vi "Send command.vi"(3 "Value":u16, 4 "Command":T1=17 items=["Measured main TEC temperature"=0, "Measured SHG heater temperature"=1, "Measured BRF heater temperature"=2, "Main TEC temperature command"=3, "SHG heater temperature command"=4, "BRF heater temperature command"=5, "Main TEC drive"=6, "SHG heater drive"=7, "BRF heater drive"=8, "Output power from photodiode"=9, "Output power setpoint (Get)"=10, "Output power setpoint (Set)"=11, "Start-up power setting (Get)"=12, "Start-up power setting (Set)"=13, "Measured LDD current"=14, "Maximum LDD current limit"=15, "16-bit fault code"=16, "Head serial number"=17, "Head board rev"=18, "Head type"=19, "LDD enable state"=20, "Key switch command (Get)"=24, "Key switch command (Set)"=25, "Key switch actual"=26, "Interlock status"=27, "Head hours"=28, "Photo or current mode command (Get)"=29, "Photo or current mode command (Set)"=30, "Photo or current mode actual"=31, "Analog input enable command (Get)"=32, "Analog input enable command (Set)"=33, "Analog input actual"=34, "Power supply glue input"=36, "Power supply glue output"=37], 5 "Device handle":u32) -> (0 "Error":errorcluster, 1 "response value":sgl, 2 "response":string)   [LabVIEW 2014]
uses:
  Commands.ctl
  Coherent global.vi
panel:
  # "PN 06/11/2014"
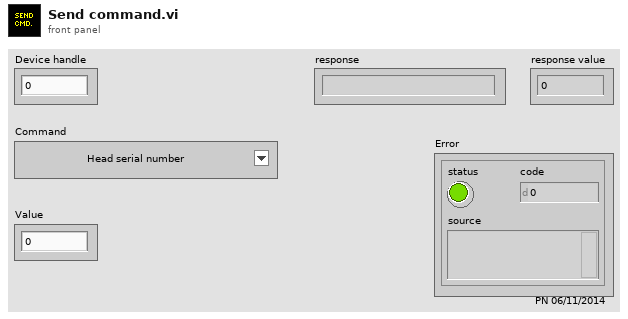
[diagram p1: front panel]
types:
  T1 = typedef "Commands.ctl" = u8
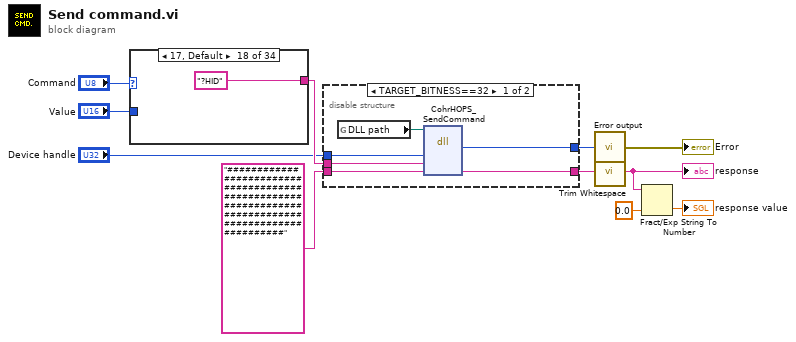
[diagram p0: block diagram]
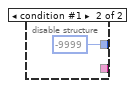
[diagram p2: hidden frame]
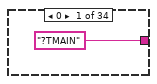
[diagram p3: hidden frame]
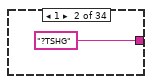
[diagram p4: hidden frame]
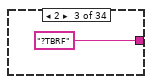
[diagram p5: hidden frame]
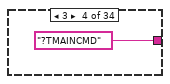
[diagram p6: hidden frame]
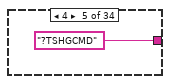
[diagram p7: hidden frame]
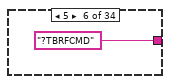
[diagram p8: hidden frame]
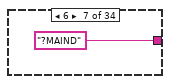
[diagram p9: hidden frame]
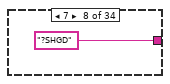
[diagram p10: hidden frame]
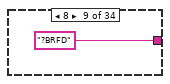
[diagram p11: hidden frame]
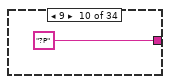
[diagram p12: hidden frame]
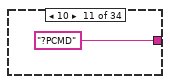
[diagram p13: hidden frame]
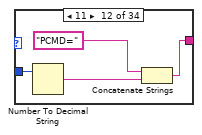
[diagram p14: hidden frame]
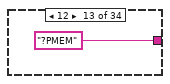
[diagram p15: hidden frame]
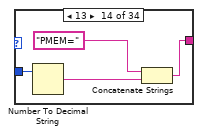
[diagram p16: hidden frame]
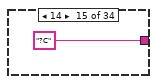
[diagram p17: hidden frame]
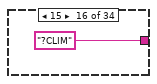
[diagram p18: hidden frame]
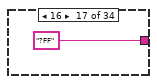
[diagram p19: hidden frame]
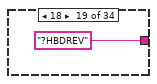
[diagram p20: hidden frame]
diagram:
  n1 = case shown="17, Default" "Command" {
    tunnel: ["?TMAIN" "?TSHG" "?TBRF" "?TMAINCMD" "?TSHGCMD" "?TBRFCMD" "?MAIND" "?SHGD" "?BRFD" "?P" "?PCMD" w23 "?PMEM" w28 "?C" "?CLIM" "?FF" "?HID" "?HBDREV" "?HTYPE" "?L" "?KSWCMD" w41 "?KSW" "?INT" "?HH" "?CMODECMD" w49 "?CMODE" "?ANACMD" w55 "?ANA" "?PSGLUEIN" "?PSGLUEOUT"] -> w9
    tunnel: "Value" -> [_ _ _ _ _ _ _ _ _ _ _ w26 _ w31 _ _ _ _ _ _ _ _ w43 _ _ _ _ w51 _ _ w57 _ _ _]
    frame 0 {
    }
    frame 1 {
    }
    frame 2 {
    }
    frame 3 {
    }
    frame 4 {
    }
    frame 5 {
    }
    frame 6 {
    }
    frame 7 {
    }
    frame 8 {
    }
    frame 9 {
    }
    frame 10 {
    }
    frame 11 {
      n2 = Number To Decimal String(number=w26) -> (decimal integer string=w25:string)  [unwired: 1 in]
      n3 = Concatenate Strings("PCMD=", w25) -> (w23:string)
    }
    frame 12 {
    }
    frame 13 {
      n4 = Number To Decimal String(number=w31) -> (decimal integer string=w30:string)  [unwired: 1 in]
      n5 = Concatenate Strings("PMEM=", w30) -> (w28:string)
    }
    frame 14 {
    }
    frame 15 {
    }
    frame 16 {
    }
    frame 17, Default {
    }
    frame 18 {
    }
    frame 19 {
    }
    frame 20 {
    }
    frame 24 {
    }
    frame 25 {
      n6 = Number To Decimal String(number=w43) -> (decimal integer string=w40:string)  [unwired: 1 in]
      n7 = Concatenate Strings("KSWCMD=", w40) -> (w41:string)
    }
    frame 26 {
    }
    frame 27 {
    }
    frame 28 {
    }
    frame 29 {
    }
    frame 30 {
      n8 = Number To Decimal String(number=w51) -> (decimal integer string=w48:string)  [unwired: 1 in]
      n9 = Concatenate Strings("CMODECMD=", w48) -> (w49:string)
    }
    frame 31 {
    }
    frame 32 {
    }
    frame 33 {
      n10 = Number To Decimal String(number=w57) -> (decimal integer string=w54:string)  [unwired: 1 in]
      n11 = Concatenate Strings("ANACMD=", w54) -> (w55:string)
    }
    frame 34 {
    }
    frame 36 {
    }
    frame 37 {
    }
  }
  n12 = disable-structure shown="TARGET_BITNESS==32" {
    disable-tunnel: "####################################################################################################" ("headType") -> [w66 _]
    disable-tunnel: "Device handle" -> [w65 _]
    disable-tunnel: w9 -> [w64 _]
    disable-tunnel: [w63 -9999 ("return value")] -> w8
    disable-tunnel: [w62 _] -> w7
    frame condition #0 (active) {
      n13 = global read "Coherent global.vi" "DLL path"() -> (w61:path)
      n14 = dll-call lib="C:/Program Files (x86)/Coherent/HOPS/CohrHOPS.dll" fn="CohrHOPS_SendCommand"(path in=w61, "handle"=w65, "command"=w64, "response"=w66) -> ("return value"=w63:i32, "response"=w62:string)  [unwired: 4 in, 2 out]
    }
    frame condition #1 {
    }
  }
  n15 = call "Error output.vi"("I32 err code"=w8) -> ("Error Out"=→"Error":errorcluster)
  n16 = call <vilib>:"Trim Whitespace.vi"("string"=w7) -> ("trimmed string"=w3:string)  [unwired: 1 in]
  "response" <- w3
  n17 = Fract/Exp String To Number(string=w3, default (0 dbl)=sgl 0.0 ("default (0 DBL)")) -> (number=→"response value":sgl)  [unwired: 2 in, 1 out]
